vi "Center Scan calculation.vi"(2 "2D or 1D Scan":bool, 3 "Fast Scan Dir":bool, 4 "Input parameters":T1) -> (0 "X":dbl, 1 "Y":dbl)   [LabVIEW 2014]
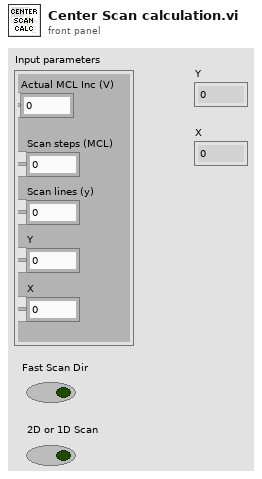
[diagram p1: front panel]
types:
  T1 = cluster{"Actual MCL Inc (V)":dbl, "Scan steps (MCL)":u64, "Scan lines (y)":u64, "Y":dbl, "X":dbl}
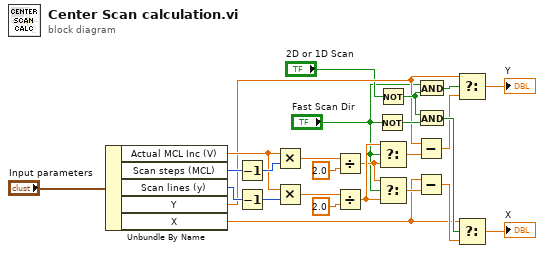
[diagram p0: block diagram]
diagram:
  n1 = Unbundle By Name("Input parameters") -> ("Actual MCL Inc (V)"=w9:dbl, "Scan steps (MCL)"=w8:u64, "Scan lines (y)"=w7:u64, "Y"=w6:dbl, "X"=w5:dbl)
  n2 = Decrement(x=w8) -> (x-1=w14:u64)
  n3 = Decrement(x=w7) -> (x-1=w12:u64)
  n4 = Multiply(x=w9, y=w14) -> (x*y=w13:dbl)
  n5 = Multiply(x=w9, y=w12) -> (x*y=w11:dbl)
  n6 = Divide(x=w13, y=2.0) -> (x/y=w17:dbl)
  n7 = Divide(x=w11, y=2.0) -> (x/y=w18:dbl)
  n8 = Not(x="Fast Scan Dir") -> (.not. x?=w22:bool)
  n9 = Not(x="2D or 1D Scan") -> (.not. x?=w23:bool)
  n10 = Select(t=w18, s="Fast Scan Dir", f=w17) -> (s? t:f=w20:dbl)
  n11 = Select(t=w17, s="Fast Scan Dir", f=w18) -> (s? t:f=w16:dbl)
  n12 = Subtract(x=w6, y=w20) -> (x-y=w19:dbl)
  n13 = Subtract(x=w5, y=w16) -> (x-y=w15:dbl)
  n14 = And(x="Fast Scan Dir", y=w23) -> (x .and. y?=w24:bool)
  n15 = And(x=w23, y=w22) -> (x .and. y?=w25:bool)
  n16 = Select(t=w6, s=w24, f=w19) -> (s? t:f=→"Y":dbl)
  n17 = Select(t=w5, s=w25, f=w15) -> (s? t:f=→"X":dbl)
